vi "ex_CheckAllT0DtEqualAttr.vi"(1 "Attributes":T1[](array[typedef]) {"dX" format="%.2f"; "X0" format="%<%X\n%x>T"; "Timestamp" format="%<%X\n%x>T"; "Start Timestamp" format="%<%X\n%x>T"}) -> (0 "All dt and t0 equal?":bool)   [LabVIEW 2017]
uses:
  <vilib>/express/express shared/transition.llb/ex_WaveformAttribsPlus.ctl
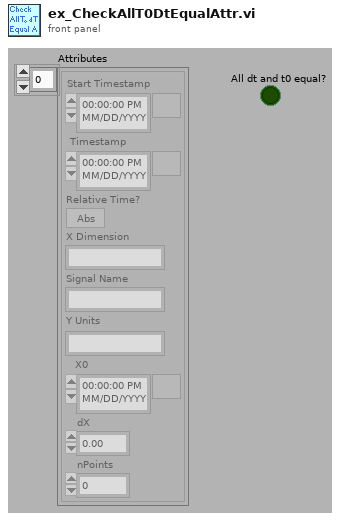
[diagram p1: front panel]
types:
  T1 = typedef "ex_WaveformAttribsPlus.ctl" = cluster{"Start Timestamp":timestamp, "Timestamp":timestamp, "Relative Time?":bool, "X Dimension":string, "Signal Name":string, "Y Units":string, "X0":timestamp, "dX":dbl, "nPoints":i32}
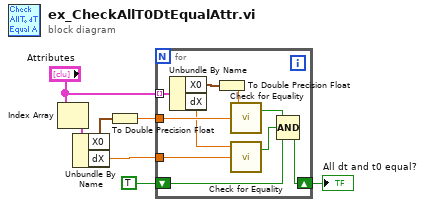
[diagram p0: block diagram]
diagram:
  n1 = Index Array(array="Attributes") -> (element=w4:T1)  [unwired: 1 in]
  n2 = Unbundle By Name(w4) -> ("X0"=w2:timestamp, "dX"=w3:dbl)
  n3 = To Double Precision Float(number=w2) -> (double precision float=w1:dbl)
  n4 = for {
    tunnel: "Attributes" -> [w10] mode=indexing
    shift-right: [w14] -> w6
    shift-left: TRUE -> [w13]
    tunnel: w1 -> [w17]
    tunnel: w3 -> [w15]
    n5 = Unbundle By Name(w10) -> ("X0"=w8:timestamp, "dX"=w16:dbl)
    n6 = To Double Precision Float(number=w8) -> (double precision float=w9:dbl)
    n7 = call <vilib>:"Check for Equality.vi"("n2"=w17, "n1"=w9) -> ("equal?"=w11:bool)  [unwired: 2 out]
    n8 = call <vilib>:"Check for Equality.vi"("n2"=w15, "n1"=w16) -> ("equal?"=w12:bool)  [unwired: 2 out]
    n9 = Compound Arithmetic op=AND(w11, w12, w13) -> (w14:bool)
  }
  "All dt and t0 equal?" <- w6
